vi "Initialize circuit.vi"() -> (5 "N":i32=2, 9 "Circuit cluster":T1)   [LabVIEW 2016]
uses:
  TypeDefs/Circuit Cluster.ctl
  Classes/GateAbst/GateAbst.lvclass
  Classes/Gate-UE/G-UE.lvclass
  C:/Users/Murtaza/OneDrive/LabVIEW/QuVI 2016/Classes/GateAbst/GateAbst.lvclass
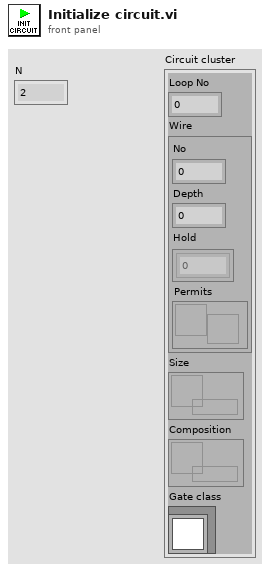
[diagram p1: front panel]
types:
  T1 = typedef "Circuit Cluster.ctl" = cluster{"Loop No":i32, "Wire":cluster{"No":i32, "Depth":i32, "Hold":i32[][], "Permits":refnum<notifier>}, "Size":refnum<queue>, "Composition":refnum<queue>, "Gate class":refnum<class "GateAbst.lvclass">}
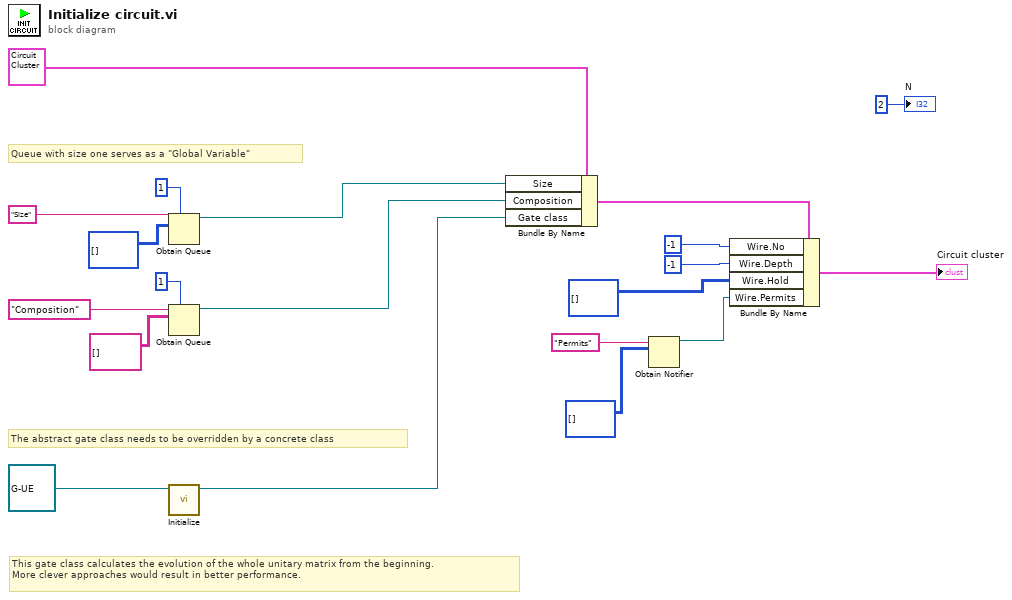
[diagram p0: block diagram]
diagram:
  # "This gate class calculates the evolution of the whole unitary matrix from the beginning. \nMore clever approaches would result in better performance."
  # "The abstract gate class needs to be overridden by a concrete class"
  # "Queue with size one serves as a \"Global Variable\""
  n1 = Obtain Queue(max queue size (-1, unlimited)=1, name (unnamed)="Size", element data type=i32[][] [] ("# Qubits")) -> (queue out=w1:refnum<queue>)  [unwired: 2 in, 2 out]
  n2 = Obtain Queue(max queue size (-1, unlimited)=1, name (unnamed)="Composition", element data type=string[][] [] ("appended array")) -> (queue out=w10:refnum<queue>)  [unwired: 2 in, 2 out]
  n3 = call-dynamic "Initialize.vi"("G-UE in"=refnum<class "G-UE.lvclass"> refnum ("G-UE.lvclass")) -> ("G-UE out"=w19:refnum<class "G-UE.lvclass">)  [unwired: 9 in, 1 out]
  n4 = Bundle By Name(cluster=T1 {"Loop No"=0, "Wire"={"No"=0, "Depth"=0, "Hold"=[], "Permits"=refnum}, "Size"=refnum, "Composition"=refnum, "Gate class"=refnum} ("Circuit cluster"), "Size"=w1, "Composition"=w10, "Gate class"=w19) -> (w9:T1)
  n5 = Obtain Notifier(name (unnamed)="Permits", notification data type=i32[][] []) -> (notifier out=w2:refnum<notifier>)  [unwired: 2 in, 2 out]
  n6 = Bundle By Name(cluster=w9, "Wire.No"=-1 ("Wire Number"), "Wire.Depth"=-1 ("Wire No"), "Wire.Hold"=i32[][] [], "Wire.Permits"=w2) -> (→"Circuit cluster":T1)
  "N" <- 2 ("N")
